vi "Set FPGA Int.vi"(0 "reference in":refnum<class "PM_Group.lvclass">, 1 "FPGA API":refnum<class "FPGA API.lvclass">) -> (14 "reference out":refnum<class "PM_Group.lvclass">)   [LabVIEW 2019, in "PM_Group.lvclass"]
uses:
  PM_Group.lvclass
  FPGA_API_class/FPGA API.lvclass
  PM_Group.lvclass/PM_Group.ctl
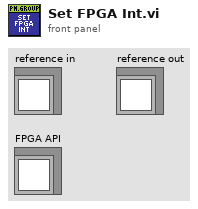
[diagram p1: front panel]
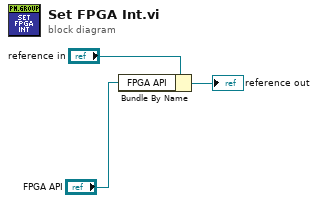
[diagram p0: block diagram]
diagram:
  n1 = Bundle By Name(cluster="reference in", "FPGA API"="FPGA API") -> (→"reference out":refnum<class "PM_Group.lvclass">)
